vi "Module Type.vi"(11 "Status Submodule in":refnum<class "Status Submodule.lvclass">) -> (2 "Module Type":string)   [LabVIEW 2020, in "VolatusSeq.lvlib" / "Status Submodule.lvclass"]
uses:
  Status Submodule.lvclass
  Status Submodule.lvclass/Status Submodule.ctl
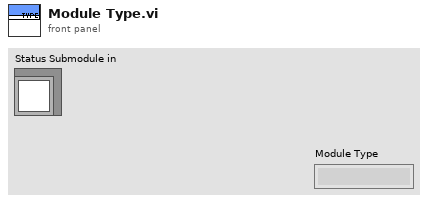
[diagram p1: front panel]
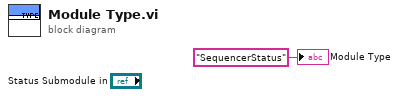
[diagram p0: block diagram]
diagram:
  "Module Type" <- "SequencerStatus" ("Module Type")
